vi "Configure Current1.vi"(6 "Current Integration Time (10: 10)":dbl(ring)=10.0 items=["0.02"=0.02, "0.2"=0.2, "1"=1.0, "10"=10.0, "100"=100.0], 7 "Terminal Type (3: 3 A Terminal)":i32(ring)=3 items=["3 A Terminal"=3, "10 A Terminal"=10], 8 "error in (no error)":errorcluster, 9 "Current Type (0: AC)":i32(ring) items=["AC", "DC"], 10 "Current Bandwidth (20 Hz)":dbl(ring)=20.0 items=["3"=3.0, "20"=20.0, "200"=200.0], 11 "VISA resource name":refnum<visa-resource-name>) -> (0 "error out":errorcluster, 3 "VISA resource name out":refnum<visa-resource-name>)   [LabVIEW 2015, in "Agilent 3446X Series1.lvlib"]
doc: "Configures current settings."
uses:
  Agilent 3446X Series1.lvlib
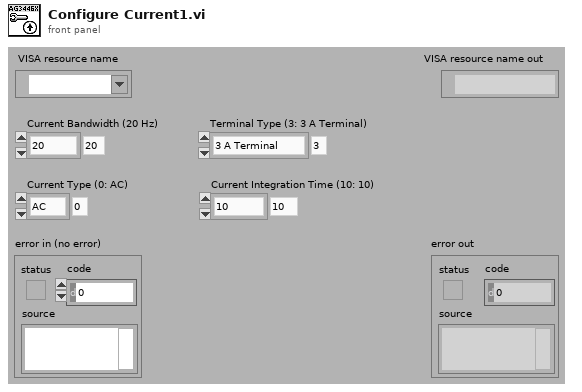
[diagram p1: front panel]
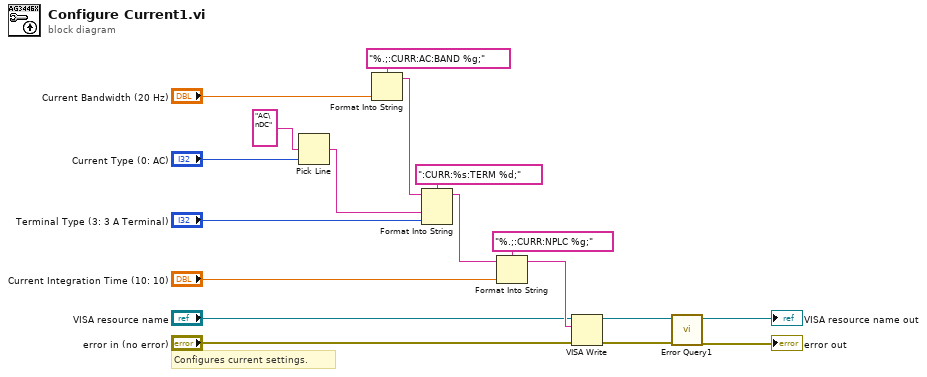
[diagram p0: block diagram]
diagram:
  # "Configures current settings."
  n1 = Pick Line(multi-line string="AC\nDC", line index="Current Type (0: AC)") -> (output string=w12:string)  [unwired: 1 out]
  n2 = Format Into String(format string="%.;:CURR:AC:BAND %g;", "Current Bandwidth (20 Hz)") -> (resulting string=w14:string)  [unwired: 2 in, 1 out]
  n3 = Format Into String(format string=":CURR:%s:TERM %d;", initial string=w14, w12, "Terminal Type (3: 3 A Terminal)") -> (resulting string=w10:string)  [unwired: 1 in, 1 out]
  n4 = Format Into String(format string="%.;:CURR:NPLC %g;", initial string=w10, "Current Integration Time (10: 10)") -> (resulting string=w7:string)  [unwired: 1 in, 1 out]
  n5 = VISA Write(VISA resource name="VISA resource name", write buffer=w7, error in (no error)="error in (no error)") -> (VISA resource name out=w4:refnum<visa-resource-name>, error out=w3:errorcluster)  [unwired: 1 out]
  n6 = call "Error Query1.vi"("error in (no error)"=w3, "VISA resource name"=w4) -> ("error out"=→"error out":errorcluster, "VISA resource name out"=→"VISA resource name out":refnum<visa-resource-name>)  [unwired: 8 out]
